vi "Write Read Process.vi"(8 "error in (no error)":errorcluster, 9 "Responce Bytes Count Required":u32, 10 "Request":string, 11 "VISA Refnum in":refnum<visa-resource-name>) -> (0 "error out":errorcluster, 1 "Responce Byted Count Returned":u32, 2 "Responce":string, 3 "VISA Refnum out":refnum<visa-resource-name>)   [LabVIEW 2017, in "Samwontech TEMP2xxx.lvlib"]
uses:
  <instrlib>/Samwontech TEMP2xxx/Samwontech TEMP2xxx.lvlib
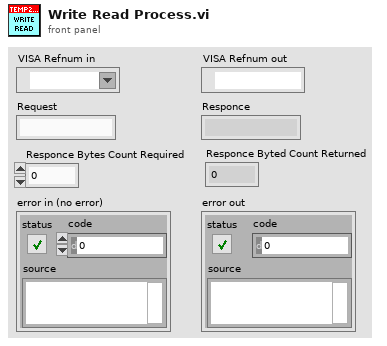
[diagram p1: front panel]
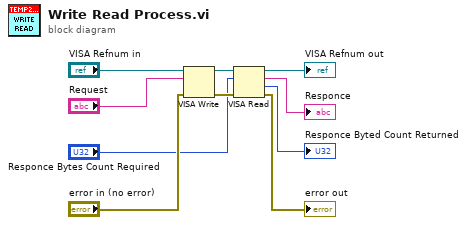
[diagram p0: block diagram]
diagram:
  n1 = VISA Write(VISA resource name="VISA Refnum in", write buffer="Request", error in (no error)="error in (no error)") -> (VISA resource name out=w4:refnum<visa-resource-name>, error out=w3:errorcluster)  [unwired: 1 out]
  n2 = VISA Read(VISA resource name=w4, byte count="Responce Bytes Count Required", error in (no error)=w3) -> (VISA resource name out=→"VISA Refnum out":refnum<visa-resource-name>, read buffer=→"Responce":string, return count=→"Responce Byted Count Returned":u32, error out=→"error out":errorcluster)
